vi "Get PID Configuration.vi"(8 "error in (no error)":errorcluster, 11 "Connection Info":T3) -> (0 "error out":errorcluster, 1 "Timed Out?":bool, 2 "Settings":T1, 3 "Connection Info Out":T3)   [LabVIEW 2013, in "PID Control Host API.lvlib"]
uses:
  PID Control Host API.lvlib
  <userlib>/STM/TCP/stm_TCP Connection Info.ctl
  <userlib>/STM/_SubVIs/stm_MetaDataElement.ctl
  Shared/Types/Get Settings Message.ctl
  Shared/Types/Gain Schedule.ctl
  Shared/Control Addon Shared.lvlib
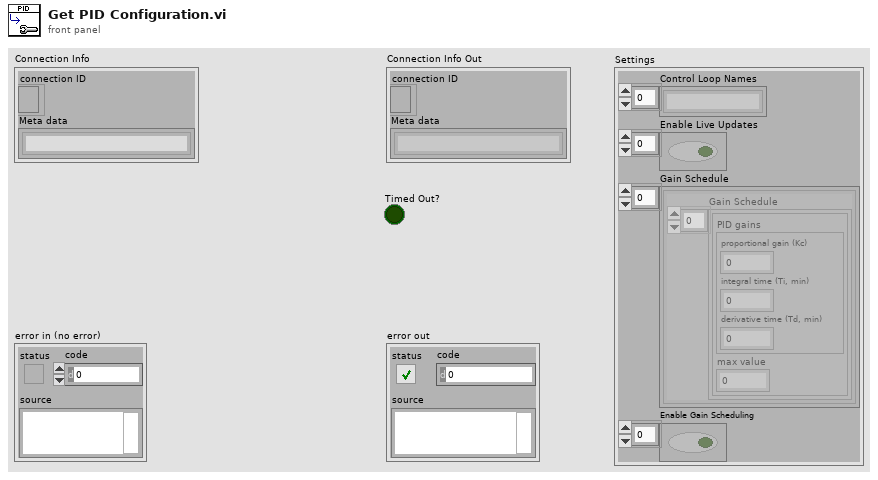
[diagram p1: front panel]
types:
  T1 = typedef "Control Addon Shared.lvlib/Get Settings Message.ctl" = cluster{"Control Loop Names":string[], "Enable Live Updates":bool[], "Gain Schedule":T2[], "Enable Gain Scheduling":bool[]}
  T2 = typedef "Control Addon Shared.lvlib/Gain Schedule.ctl" = cluster{"Gain Schedule":cluster{"PID gains":cluster{"proportional gain (Kc)":dbl, "integral time (Ti, min)":dbl, "derivative time (Td, min)":dbl}, "max value":dbl}[]}
  T3 = typedef "stm_TCP Connection Info.ctl" = cluster{"connection ID":refnum<k5>, "Meta data":T4[]}
  T4 = typedef "stm_MetaDataElement.ctl" = string
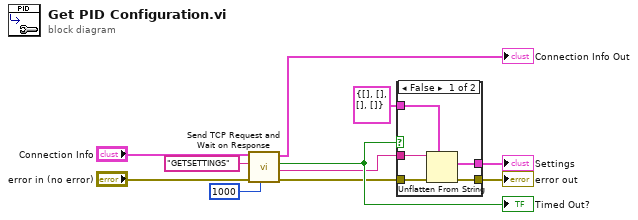
[diagram p0: block diagram]
diagram:
  n1 = call "Send TCP Request and Wait on Response.vi"("Timeout (ms)"=u32 1000, "error in (no error)"="error in (no error)", "Name"="GETSETTINGS", "Connection Info"="Connection Info") -> ("error out"=w5:errorcluster, "Data"=w4:string, "Timed Out?"=w7:bool, "Connection Info Out"=→"Connection Info Out":T3)  [unwired: 4 in]
  "Timed Out?" <- w7
  n2 = case shown="False" w7 {
    tunnel: w4 -> [w16 _]
    tunnel: w5 -> [w15 w18]
    tunnel: [w14 w18] -> w3
    tunnel: [w13 w17] -> w2
    tunnel: T1 {"Control Loop Names"=[], "Enable Live Updates"=[], "Gain Schedule"=[], "Enable Gain Scheduling"=[]} ("GetSettings") -> [w12 w17]
    frame False {
      n3 = Unflatten From String(type=w12, binary string=w16, error in (no error)=w15) -> (value=w13:T1, error out=w14:errorcluster)  [unwired: 2 in, 1 out]
    }
    frame True {
    }
  }
  "error out" <- w3
  "Settings" <- w2
